vi "All Sensor Values.vi"() -> ()   [LabVIEW 2013]
uses:
  Globals/Useful Values.vi
  Globals/Data for Dashboard.vi
panel:
  out "Interposer Pot":dbl
  out "Arm Pot vs Setpoint":cluster{"Voltage":dbl, "Angle":dbl}(graph)
  out "Winch Sensor":bool
  out "Ball Sensor":bool
  out "Right Distance":dbl
  out "Left Distance":dbl
  out "Intake":dbl
  out "Jew Bar":dbl
  out "Roller":dbl
  out "Trigger":dbl
  out "Winch":dbl
  out "Arm":dbl
  out "Right Drive":dbl
  out "Left Drive":dbl
  out "Winch Limit Switch":bool
  out "Trigger Limit Switch":bool
  out "Intake Pot":dbl
  out "Winch Pot":dbl
  out "Arm Pot":dbl
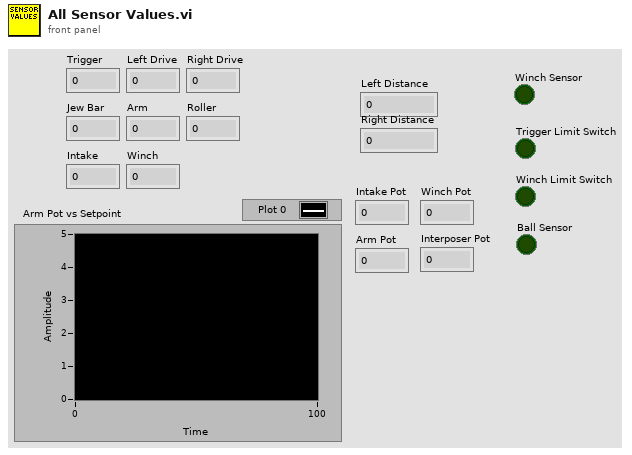
[diagram p1: front panel]
types:
  T1 = typedef "WPI_EncoderDevRef.ctl" = cluster{"DevStatus":errorcluster, "EncoderIndex":T2, "CounterIndex":T3, "DistancePerCount":dbl, "Decoding Type":T4}
  T2 = typedef "FPGA_EncoderIdx.ctl" = enum8{"Enc 0", "Enc 1", "Enc 2", "Enc 3", "Invalid"}
  T3 = typedef "FPGA_CounterCtrSystemIndex.ctl" = enum8{"Ctr 0", "Ctr 1", "Ctr 2", "Ctr 3", "Ctr 4", "Ctr 5", "Ctr 6", "Ctr 7", "Invalid"}
  T4 = typedef "WPI_EncoderType.ctl" = enum16{"1x", "2x", "4x"}
  T5 = typedef "WPI_MotorControlDeviceRef.ctl" = cluster{"DeviceStatus":errorcluster, "Type":enum16{"PWM", "CAN"}, "PWM":cluster{"Digital Module":T6, "PWM Channel":T7, "DeadBand":T8}, "CAN":cluster{"Device Number":u8, "Control Mode":T9, "Semaphore":T10, "Max Vout":dbl}, "Invert":bool, "TransformRef":T11, "InvTransformRef":T11}
  T6 = typedef "FPGA_TypedefDigitalModule.ctl" = enum16{"Digital Module 1", "Digital Module 2"}
  T7 = typedef "FPGA_DIOPWMChannel.ctl" = enum8{"PWM 1", "PWM 2", "PWM 3", "PWM 4", "PWM 5", "PWM 6", "PWM 7", "PWM 8", "PWM 9", "PWM 10", "Invalid"}
  T8 = typedef "WPI_PWMDeadband.ctl" = cluster{"Name":string, "maxPositivePwm":i32, "minPositivePwm":i32, "centerPwm":i32, "maxNegativePwm":i32, "minNegativePwm":i32, "angularRange":u16}
  T9 = typedef "WPI_CANJaguar_ControlMode.ctl" = enum8{"Percent VBus", "Current", "Speed", "Position", "Voltage"}
  T10 = typedef "Semaphore RefNum" = refnum<k1>
  T11 = typedef "WPI_PWMTransform_ConPane.ctl" = refnum<vi>
  T12 = typedef "WPI_DigitalInputDevRef.ctl" = cluster{"DevStatus":errorcluster, "DIO Channel":T13, "Digital Module":T6}
  T13 = typedef "FPGA_DIOChannel.ctl" = enum8{"DIO 1", "DIO 2", "DIO 3", "DIO 4", "DIO 5", "DIO 6", "DIO 7", "DIO 8", "DIO 9", "DIO 10", "DIO 11", "DIO 12", "DIO 13", "DIO 14", "Invalid"}
  T14 = typedef "WPI_AnalogChannelDevRef.ctl" = cluster{"DevStatus":errorcluster, "Analog Module":T15, "Analog Channel":T16}
  T15 = typedef "FPGA_TypedefAnalogModule.ctl" = enum16{"Analog Module 1", "Analog Module 2"}
  T16 = typedef "FPGA_AIChannel.ctl" = enum8{"AI 1", "AI 2", "AI 3", "AI 4", "AI 5", "AI 6", "AI 7", "AI 8", "Invalid"}
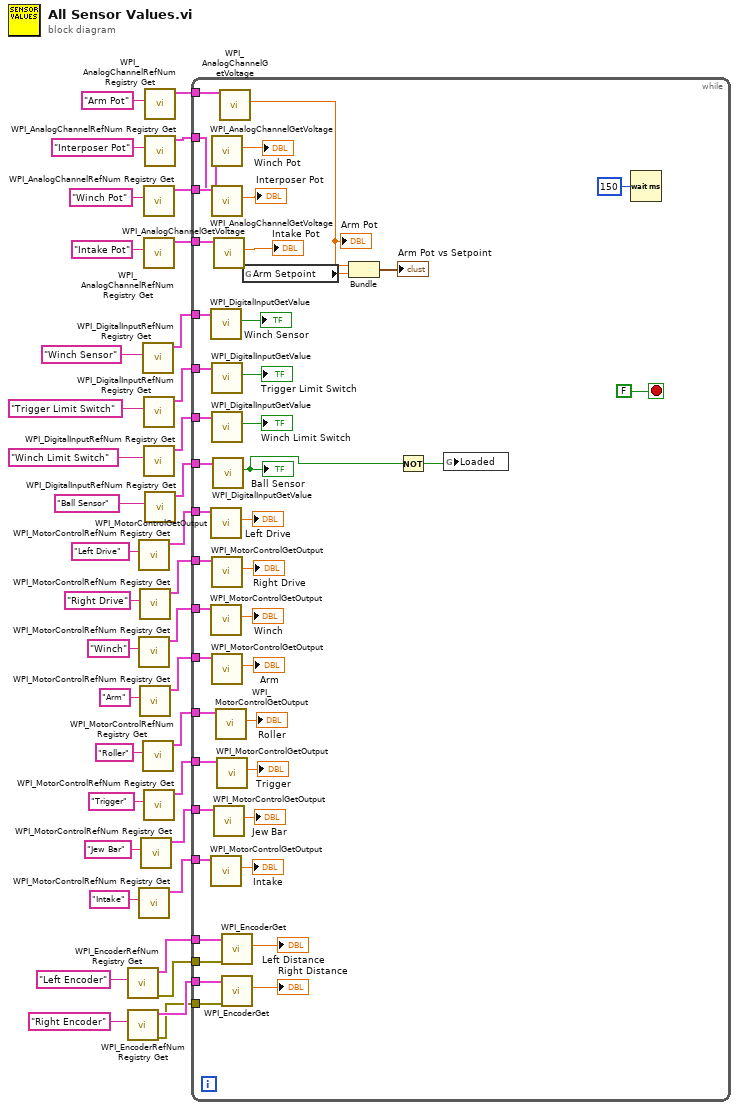
[diagram p0: block diagram]
diagram:
  n1 = call <vilib>:"WPI_EncoderRefNum Registry Get.vi"("refnum name"="Left Encoder") -> ("error out"=w12:errorcluster, "EncoderDevRef"=w11:T1)  [unwired: 9 in]
  n2 = call <vilib>:"WPI_EncoderRefNum Registry Get.vi"("refnum name"="Right Encoder") -> ("error out"=w7:errorcluster, "EncoderDevRef"=w8:T1)  [unwired: 9 in]
  n3 = call <vilib>:"WPI_MotorControlRefNum Registry Get.vi"("refnum name"="Left Drive") -> ("MotorControlDevRef"=w28:T5)  [unwired: 9 in, 1 out]
  n4 = call <vilib>:"WPI_MotorControlRefNum Registry Get.vi"("refnum name"="Winch") -> ("MotorControlDevRef"=w21:T5)  [unwired: 9 in, 1 out]
  n5 = call <vilib>:"WPI_MotorControlRefNum Registry Get.vi"("refnum name"="Intake") -> ("MotorControlDevRef"=w14:T5)  [unwired: 9 in, 1 out]
  n6 = call <vilib>:"WPI_MotorControlRefNum Registry Get.vi"("refnum name"="Right Drive") -> ("MotorControlDevRef"=w25:T5)  [unwired: 9 in, 1 out]
  n7 = call <vilib>:"WPI_MotorControlRefNum Registry Get.vi"("refnum name"="Arm") -> ("MotorControlDevRef"=w24:T5)  [unwired: 9 in, 1 out]
  n8 = call <vilib>:"WPI_MotorControlRefNum Registry Get.vi"("refnum name"="Jew Bar") -> ("MotorControlDevRef"=w15:T5)  [unwired: 9 in, 1 out]
  n9 = call <vilib>:"WPI_DigitalInputRefNum Registry Get.vi"("refnum name"="Winch Sensor") -> ("DigitalInputDevRef"=w3:T12)  [unwired: 9 in, 1 out]
  n10 = call <vilib>:"WPI_MotorControlRefNum Registry Get.vi"("refnum name"="Roller") -> ("MotorControlDevRef"=w20:T5)  [unwired: 9 in, 1 out]
  n11 = call <vilib>:"WPI_AnalogChannelRefNum Registry Get.vi"("refnum name"="Winch Pot") -> ("AIDeviceRef"=w35:T14)  [unwired: 9 in, 1 out]
  n12 = call <vilib>:"WPI_AnalogChannelRefNum Registry Get.vi"("refnum name"="Intake Pot") -> ("AIDeviceRef"=w34:T14)  [unwired: 9 in, 1 out]
  n13 = call <vilib>:"WPI_DigitalInputRefNum Registry Get.vi"("refnum name"="Trigger Limit Switch") -> ("DigitalInputDevRef"=w32:T12)  [unwired: 9 in, 1 out]
  n14 = call <vilib>:"WPI_DigitalInputRefNum Registry Get.vi"("refnum name"="Winch Limit Switch") -> ("DigitalInputDevRef"=w29:T12)  [unwired: 9 in, 1 out]
  n15 = call <vilib>:"WPI_MotorControlRefNum Registry Get.vi"("refnum name"="Trigger") -> ("MotorControlDevRef"=w17:T5)  [unwired: 9 in, 1 out]
  n16 = call <vilib>:"WPI_AnalogChannelRefNum Registry Get.vi"("refnum name"="Arm Pot") -> ("AIDeviceRef"=w38:T14)  [unwired: 9 in, 1 out]
  n17 = call <vilib>:"WPI_AnalogChannelRefNum Registry Get.vi"("refnum name"="Interposer Pot") -> ("AIDeviceRef"=w1:T14)  [unwired: 9 in, 1 out]
  n18 = call <vilib>:"WPI_DigitalInputRefNum Registry Get.vi"("refnum name"="Ball Sensor") -> ("DigitalInputDevRef"=w6:T12)  [unwired: 9 in, 1 out]
  n19 = while {
    tunnel: w38 -> [w79]
    tunnel: w35 -> [w77]
    tunnel: w34 -> [w76]
    tunnel: w32 -> [w74]
    tunnel: w29 -> [w71]
    tunnel: w28 -> [w70]
    tunnel: w25 -> [w67]
    tunnel: w21 -> [w63]
    tunnel: w24 -> [w66]
    tunnel: w20 -> [w62]
    tunnel: w17 -> [w59]
    tunnel: w15 -> [w57]
    tunnel: w14 -> [w56]
    tunnel: w12 -> [w54]
    tunnel: w11 -> [w53]
    tunnel: w7 -> [w51]
    tunnel: w8 -> [w52]
    tunnel: w6 -> [w48]
    tunnel: w3 -> [w44]
    tunnel: w1 -> [w40]
    stop <- FALSE stop-if-true
    n20 = call <vilib>:"WPI_DigitalInputGetValue.vi"("DigitalInputDevRef"=w44) -> ("Value"=→"Winch Sensor":bool)  [unwired: 8 in, 2 out]
    n21 = call <vilib>:"WPI_MotorControlGetOutput.vi"("MotorControlDevRef"=w70) -> ("Output"=→"Left Drive":dbl)  [unwired: 8 in, 2 out]
    n22 = call <vilib>:"WPI_MotorControlGetOutput.vi"("MotorControlDevRef"=w63) -> ("Output"=→"Winch":dbl)  [unwired: 8 in, 2 out]
    n23 = call <vilib>:"WPI_MotorControlGetOutput.vi"("MotorControlDevRef"=w56) -> ("Output"=→"Intake":dbl)  [unwired: 8 in, 2 out]
    n24 = call <vilib>:"WPI_AnalogChannelGetVoltage.vi"("AIDeviceRef"=w77) -> ("Voltage"=→"Winch Pot":dbl)  [unwired: 8 in, 2 out]
    n25 = call <vilib>:"WPI_AnalogChannelGetVoltage.vi"("AIDeviceRef"=w40) -> ("Voltage"=→"Interposer Pot":dbl)  [unwired: 8 in, 2 out]
    n26 = call <vilib>:"WPI_DigitalInputGetValue.vi"("DigitalInputDevRef"=w74) -> ("Value"=→"Trigger Limit Switch":bool)  [unwired: 8 in, 2 out]
    n27 = call <vilib>:"WPI_DigitalInputGetValue.vi"("DigitalInputDevRef"=w71) -> ("Value"=→"Winch Limit Switch":bool)  [unwired: 8 in, 2 out]
    n28 = call <vilib>:"WPI_MotorControlGetOutput.vi"("MotorControlDevRef"=w67) -> ("Output"=→"Right Drive":dbl)  [unwired: 8 in, 2 out]
    n29 = call <vilib>:"WPI_MotorControlGetOutput.vi"("MotorControlDevRef"=w66) -> ("Output"=→"Arm":dbl)  [unwired: 8 in, 2 out]
    n30 = call <vilib>:"WPI_DigitalInputGetValue.vi"("DigitalInputDevRef"=w48) -> ("Value"=w46:bool)  [unwired: 8 in, 2 out]
    "Ball Sensor" <- w46
    n31 = call <vilib>:"WPI_AnalogChannelGetVoltage.vi"("AIDeviceRef"=w76) -> ("Voltage"=→"Intake Pot":dbl)  [unwired: 8 in, 2 out]
    n32 = call <vilib>:"WPI_MotorControlGetOutput.vi"("MotorControlDevRef"=w57) -> ("Output"=→"Jew Bar":dbl)  [unwired: 8 in, 2 out]
    n33 = call <vilib>:"WPI_MotorControlGetOutput.vi"("MotorControlDevRef"=w62) -> ("Output"=→"Roller":dbl)  [unwired: 8 in, 2 out]
    n34 = call <vilib>:"WPI_MotorControlGetOutput.vi"("MotorControlDevRef"=w59) -> ("Output"=→"Trigger":dbl)  [unwired: 8 in, 2 out]
    n35 = call <vilib>:"WPI_AnalogChannelGetVoltage.vi"("AIDeviceRef"=w79) -> ("Voltage"=w43:dbl)  [unwired: 8 in, 2 out]
    "Arm Pot" <- w43
    n36 = call <vilib>:"WPI_EncoderGet.vi"("error in (no error)"=w54, "EncoderDevRef"=w53) -> ("Distance"=→"Left Distance":dbl)  [unwired: 4 in, 5 out]
    n37 = call <vilib>:"WPI_EncoderGet.vi"("error in (no error)"=w51, "EncoderDevRef"=w52) -> ("Distance"=→"Right Distance":dbl)  [unwired: 4 in, 5 out]
    n38 = global read "Useful Values.vi" "Arm Setpoint"() -> (w42:dbl)
    n39 = Bundle("Voltage"=w43, "Arm Setpoint"=w42) -> (→"Arm Pot vs Setpoint":cluster{"Voltage":dbl, "Arm Setpoint":dbl})  [unwired: 1 in]
    n40 = Not(x=w46) -> (.not. x?=w47:bool)
    n41 = global write "Data for Dashboard.vi" "Loaded"(w47) -> ()
    n42 = Wait (ms)(milliseconds to wait=u32 150) -> ()  [unwired: 1 out]
  }
